vi "StringArray Create.vi"(8 "error in (no error)":errorcluster, 11 "String array in":string[](array[string])) -> (0 "error out":errorcluster, 3 "StringArray DVR out":refnum<data-value>)   [LabVIEW 2010, in "MDSplus.lvlib"]
uses:
  <vilib>/MDSplus/Library/MDSplus.lvlib
  <vilib>/MDSplus/Classes/Data_Class/Array_Class/StringArray_Class/StringArray.lvclass
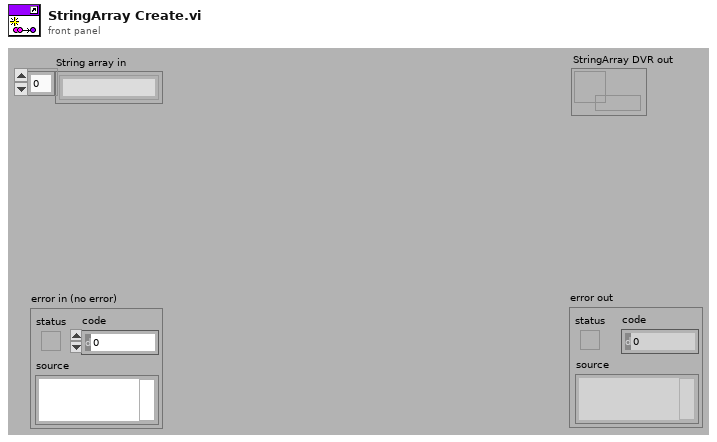
[diagram p1: front panel]
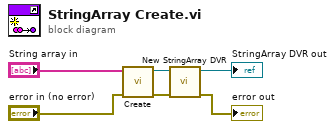
[diagram p0: block diagram]
diagram:
  n1 = call <vilib>:"Create.vi"("error in (no error)"="error in (no error)", "String array in"="String array in") -> ("error out"=w4:errorcluster, "StringArray out"=w5:refnum<class "StringArray.lvclass">)  [unwired: 8 in]
  n2 = call <vilib>:"New StringArray DVR.vi"("error in (no error)"=w4, "StringArray in"=w5) -> ("error out"=→"error out":errorcluster, "StringArray DVR out"=→"StringArray DVR out":refnum<data-value>)  [unwired: 8 in]
